vi "Start Continuous Output.vi"(8 "error in (no error)":errorcluster, 10 "time interval (1 s)":u16(ring)=1 items=["100 ms", "1 s", "1 min."], 11 "VGC in":refnum<class "PL Inficon VGC.lvclass">) -> (0 "error out":errorcluster, 3 "VGC out":refnum<class "PL Inficon VGC.lvclass">)   [LabVIEW 2015, in "PL Inficon VGC.lvclass"]
doc: "Starts continuous output of measured values."
uses:
  PL Inficon VGC.lvclass
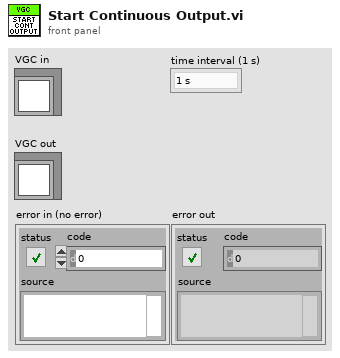
[diagram p1: front panel]
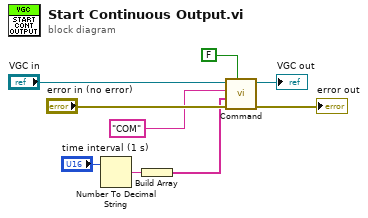
[diagram p0: block diagram]
diagram:
  n1 = Number To Decimal String(number="time interval (1 s)") -> (decimal integer string=w5:string)  [unwired: 1 in]
  n2 = Build Array(w5) -> (w4:string[])
  n3 = call "Command.vi"("receive data (true)"=FALSE, "error in (no error)"="error in (no error)", "parameters"=w4, "command"="COM", "VGC in"="VGC in") -> ("error out"=→"error out":errorcluster, "VGC out"=→"VGC out":refnum<class "PL Inficon VGC.lvclass">)  [unwired: 4 in, 1 out]
